vi "superposition.vi"() -> ()   [LabVIEW 2015]
panel:
  in  "y1":dbl
  in  "y0":dbl
  in  "d":dbl
  in  "row (px)":i32=64
  in  "col (px)":i32=64
  out "Mode":dbl[][](graph)
  out "Phase":dbl[][](graph)
  out "Intensity":dbl[][](graph)
  in  "?":bool
  in  "beam waist w0 (m)":dbl=0.0001 format="%.2p"
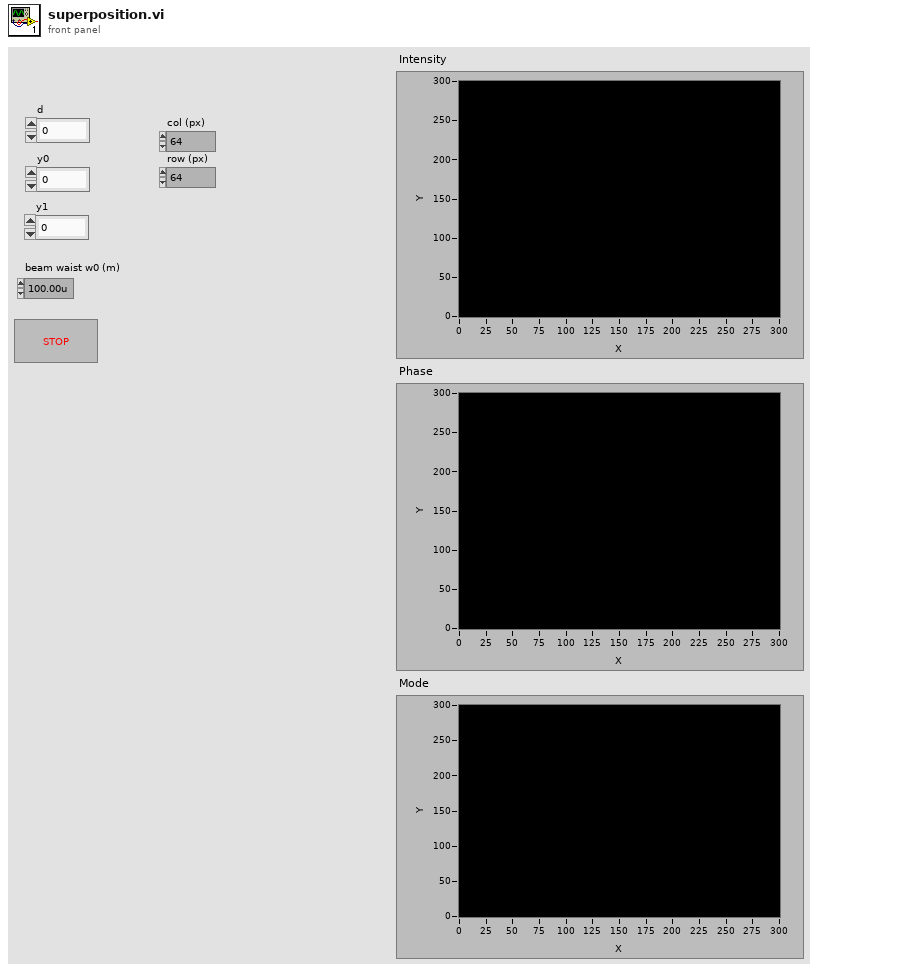
[diagram p1: front panel]
types:
  T1 = cluster{"amplitude matrix":cdb[][], "number of columns in amplitude matrix":i32, "number of rows in amplitude matrix":i32, "represented width (in m)":dbl, "represented height (in m)":dbl, "wavelength (in m)":dbl}
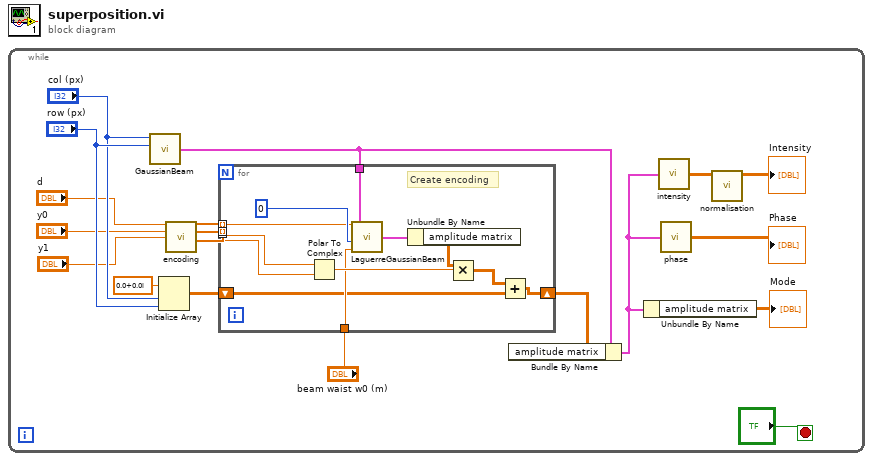
[diagram p0: block diagram]
diagram:
  n1 = while {
    stop <- "?" stop-if-true
    n2 = call <userlib>:"GaussianBeam.vi"("number of rows in amplitude matrix (default 64)"="row (px)", "number of columns in amplitude matrix (default 64)"="col (px)") -> ("Gaussian beam"=w14:T1)  [unwired: 4 in]
    n3 = Initialize Array(cdb 0.0+0.0i ("element"), "col (px)", "row (px)") -> (w17:cdb[][])
    n4 = call "encoding.vi"("d"="d", "y0"="y0", "y1"="y1") -> ("modes"=w6:dbl[], "coeffs"=w5:dbl[], "phase"=w4:dbl[])  [unwired: 10 in]
    n5 = for {
      tunnel: w14 -> [w28]
      tunnel: "beam waist w0 (m)" -> [w27]
      shift-right: [w24] -> w15
      shift-left: w17 -> [w25]
      tunnel: w6 -> [w22] mode=indexing
      tunnel: w5 -> [w20] mode=indexing
      tunnel: w4 -> [w21] mode=indexing
      # "Create encoding"
      n6 = Polar To Complex(1:w21, 2:w20) -> (0:w29:cdb)
      n7 = call <userlib>:"LaguerreGaussianBeam.vi"("beam waist w0 (in m; default 1E-4 = 0.1mm)"=w27, "p"=0, "l"=w22, "beam parameters"=w28) -> ("Laguerre-Gaussian beam"=w23:T1)
      n8 = Unbundle By Name(w23) -> ("amplitude matrix"=w30:cdb[][])
      n9 = Multiply(x=w30, y=w29) -> (x*y=w26:cdb[][])
      n10 = Add(x=w26, y=w25) -> (x+y=w24:cdb[][])
    }
    n11 = Bundle By Name(cluster=w14, "amplitude matrix"=w15) -> (w12:T1)
    n12 = Unbundle By Name(w12) -> ("amplitude matrix"=→"Mode":cdb[][])
    n13 = call <userlib>:"intensity.vi"("beam cluster"=w12) -> ("intensity matrix"=w10:dbl[][])
    n14 = call <userlib>:"phase.vi"("beam cluster"=w12) -> ("phase matrix"=→"Phase":dbl[][])
    n15 = call "normalisation.vi"("intensity matrix"=w10) -> ("Array"=→"Intensity":dbl[][])  [unwired: 10 in]
  }
